vi "Test GPU FFT.vi"() -> ()   [LabVIEW 2018]
panel:
  out "h_ret":u16[](graph)
  out "Waveform Chart":dbl(graph)
  out "time":dbl
  out "h_ref":sgl[](graph)
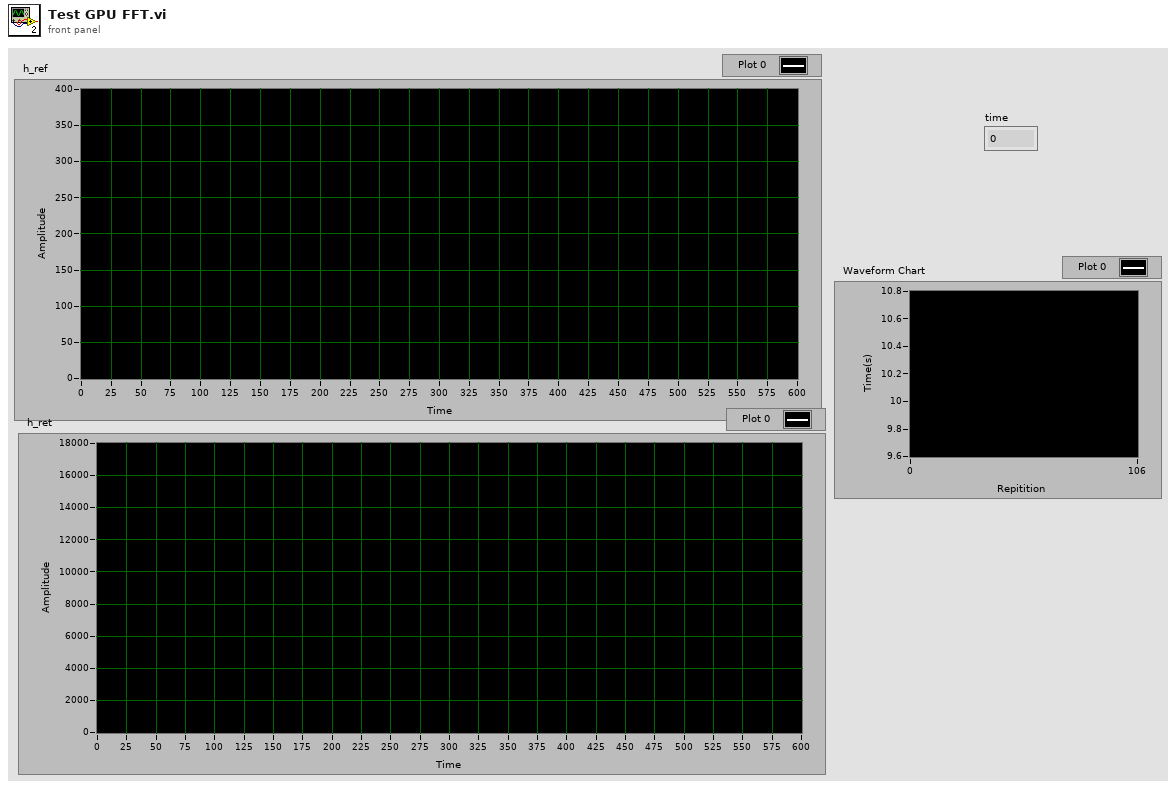
[diagram p1: front panel]
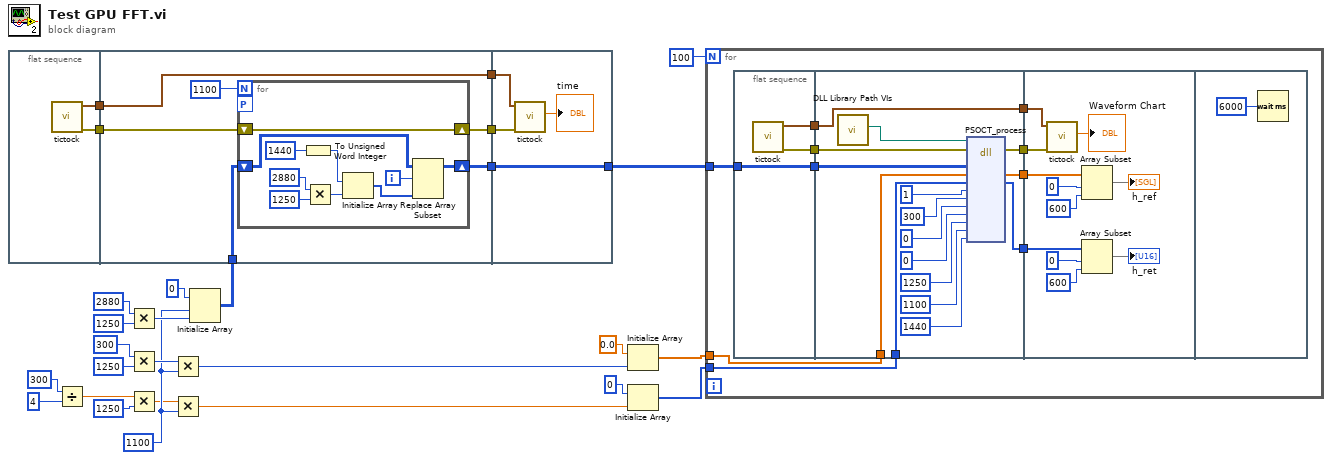
[diagram p0: block diagram]
diagram:
  w14 = 1100 ("dimension size")
  n1 = flat-sequence {
    tunnel: [w29] -> w7
    tunnel: [w28] -> w6
    tunnel: [w35] -> w5
    tunnel: w7 -> [w35]
    tunnel: w6 -> [w30]
    tunnel: [w34] -> w4
    tunnel: w2 -> [w33]
    tunnel: [w32] -> w3
    tunnel: w5 -> [w49]
    tunnel: w4 -> [w48]
    tunnel: w3 -> [w46]
    tunnel: [w46] -> w1
    frame #0 {
      n2 = call "tictock.vi"() -> ("error out"=w28:errorcluster, "seconds since 1Jan1904"=w29:timestamp)  [unwired: 9 in, 1 out]
    }
    frame #1 {
      n3 = for {
        N: 1100 ("x") -> [_]
        shift-right: [w36] -> w34
        shift-left: w30 -> [w36]
        shift-right: [w44] -> w32
        shift-left: w33 -> [w45]
        workers-P: _ -> [_]
        i -> [w43]
        n4 = To Unsigned Word Integer(number=u32 1440 ("element")) -> (unsigned 16bit integer=w38:u16)
        n5 = Multiply(x=u32 2880 ("element"), y=u32 1250 ("element")) -> (x*y=w42:u32)
        n6 = Initialize Array(w38, w42) -> (w39:u16[])
        n7 = Replace Array Subset(array=w45, new element=w39, index (row)=w43) -> (w44:u16[][])  [unwired: 1 in]
      }
    }
    frame #2 {
      n8 = call "tictock.vi"("error in (no error)"=w48, "seconds since 1Jan1904 2"=w49) -> ("Numeric"=→"time":dbl)  [unwired: 7 in, 2 out]
    }
  }
  n9 = Divide(x=300, y=4) -> (x/y=w9:dbl)
  n10 = Multiply(x=u32 2880 ("element"), y=u32 1250 ("element")) -> (x*y=w24:u32)
  n11 = Multiply(x=300, y=1250) -> (x*y=w22:i32)
  n12 = Multiply(x=w9, y=1250) -> (x*y=w12:dbl)
  n13 = Multiply(x=w22, y=w14) -> (x*y=w21:i32)
  n14 = Multiply(x=w12, y=w14) -> (x*y=w16:dbl)
  n15 = Initialize Array(u16 0 ("element"), w14, w24) -> (w2:u16[][])
  n16 = Initialize Array(sgl 0.0 ("element"), w21) -> (w17:sgl[])
  n17 = Initialize Array(u16 0 ("element"), w16) -> (w8:u16[])
  n18 = for {
    N: 100 -> [_]
    tunnel: w17 -> [w53]
    tunnel: w8 -> [w52]
    tunnel: w1 -> [w50]
    n19 = flat-sequence {
      tunnel: [w62] -> w59
      tunnel: [w61] -> w58
      tunnel: [w60] -> w57
      tunnel: w50 -> [w60]
      tunnel: w59 -> [w78]
      tunnel: w58 -> [w76]
      tunnel: w57 -> [w75]
      tunnel: w53 -> [w74]
      tunnel: [w73] -> w56
      tunnel: [w77] -> w55
      tunnel: [w78] -> w54
      tunnel: w52 -> [w71]
      tunnel: [w63] -> w51
      tunnel: w56 -> [w85]
      tunnel: w55 -> [w87]
      tunnel: w54 -> [w86]
      tunnel: w51 -> [w79]
      frame #0 {
        n20 = call "tictock.vi"() -> ("error out"=w61:errorcluster, "seconds since 1Jan1904"=w62:timestamp)  [unwired: 9 in, 1 out]
      }
      frame #1 {
        n21 = call "DLL Library Path VIs.vi"() -> ("GPU FFT birefringence simple ret"=w72:path)  [unwired: 5 in, 6 out]
        n22 = dll-call lib="C:/Project/SerialSectionOCT/SerialSectOCT/Labview Software/DLL/CUDA_FFT_single_channel.dll" fn="PSOCT_process"(path in=w72, error in=w76, "h_signal"=w75, "h_processed_ref"=w74, "h_processed_ret"=w71, "z0"=1, "depth"=300, "a"=0, "b"=0, "NALINES"=1250, "NBLINES"=1100, "SAMPLES"=1440) -> (error out=w77:errorcluster, "h_processed_ref"=w73:sgl[], "h_processed_ret"=w63:u16[])  [unwired: 10 in, 1 out]
      }
      frame #2 {
        n23 = call "tictock.vi"("error in (no error)"=w87, "seconds since 1Jan1904 2"=w86) -> ("Numeric"=→"Waveform Chart":dbl)  [unwired: 7 in, 2 out]
        n24 = Array Subset(array=w85, index=0, length=600) -> (→"h_ref":sgl[])
        n25 = Array Subset(array=w79, index=0, length=600) -> (→"h_ret":u16[])
      }
      frame #3 {
        n26 = Wait (ms)(milliseconds to wait=u32 6000) -> ()  [unwired: 1 out]
      }
    }
  }
